vi "Read All Analog Channels.vi"(7 "error in":errorcluster, 9 "Voltage Data":bool=TRUE, 10 "VISA resource name":refnum<visa-resource-name>) -> (0 "error out":errorcluster, 2 "Analog output cluster":T1, 3 "VISA resource name out":refnum<visa-resource-name>)   [LabVIEW 2020, in "BDAQ-6104.lvlib"]
uses:
  <instrlib>/BDAQ-6104/BDAQ-6104.lvlib
panel:
  out "read buffer":string
  in  "AIO Cluster":T1
  out "Volts 0":dbl
  out "Volts 1":dbl
  out "Volts 2":dbl
  out "Volts 3":dbl
  out "Volts 4":dbl
  out "Volts 5":dbl
  out "Value 0":i32
  out "Value 1":i32
  out "Vaolue 2":i32
  out "Value 3":i32
  out "Value 4":i32
  out "Value 5":i32
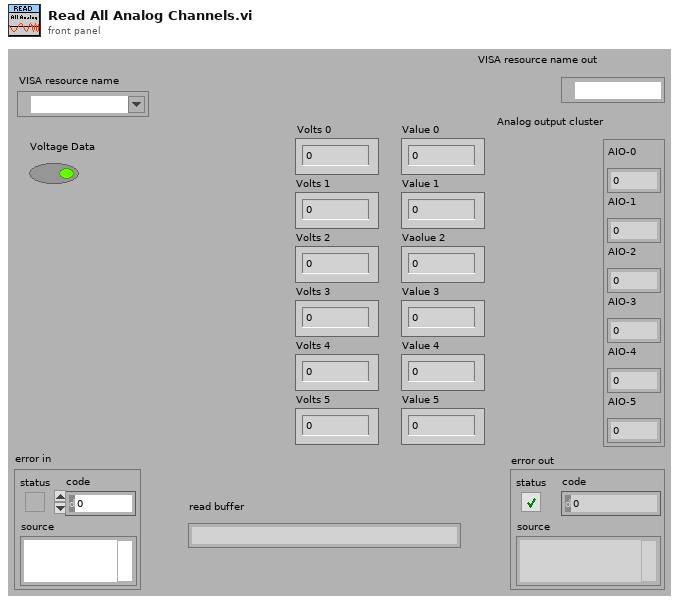
[diagram p1: front panel]
types:
  T1 = cluster{"AIO-0":dbl, "AIO-1":dbl, "AIO-2":dbl, "AIO-3":dbl, "AIO-4":dbl, "AIO-5":dbl}
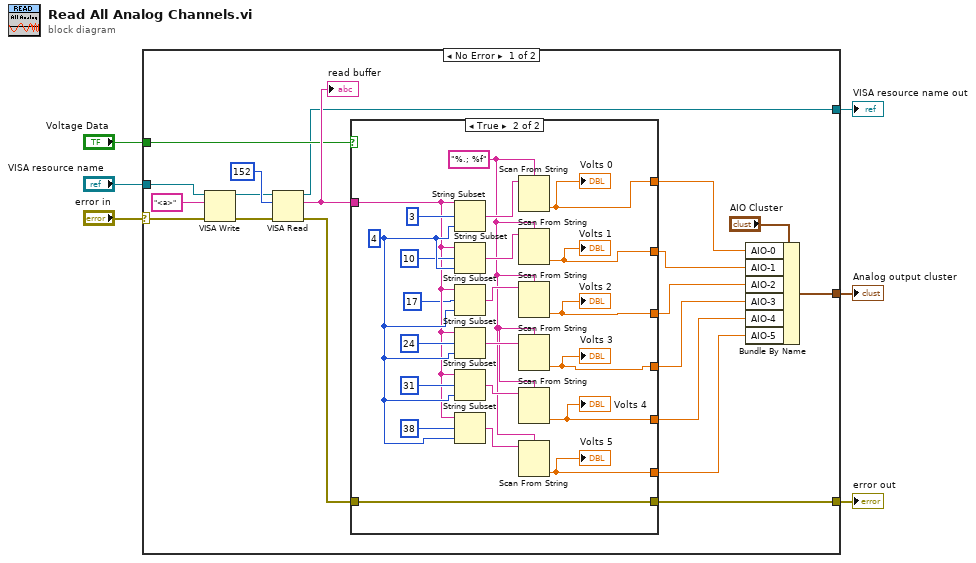
[diagram p0: block diagram]
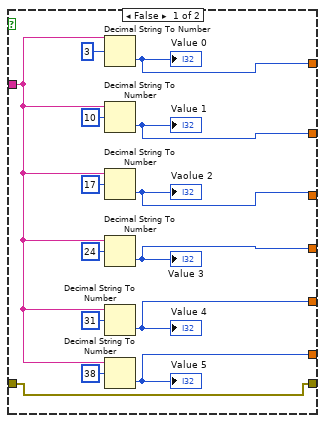
[diagram p2: hidden frame]
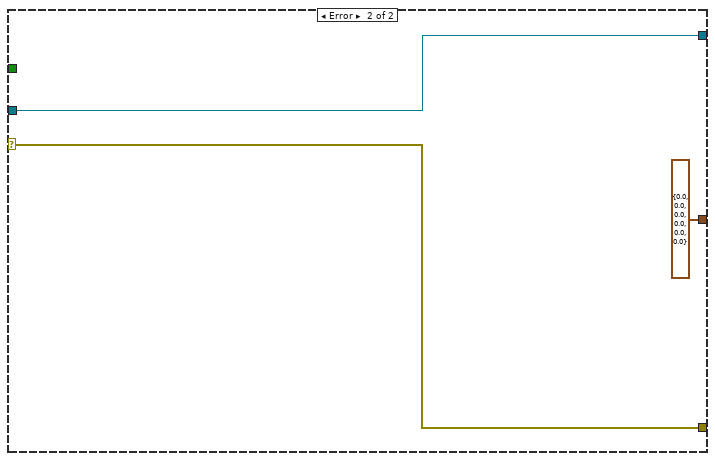
[diagram p3: hidden frame]
diagram:
  n1 = case shown="No Error" "error in" {
    selector: "error in" -> [w7 w63]
    tunnel: "VISA resource name" -> [w24 w64]
    tunnel: [w18 T1 {"AIO-0"=0.0, "AIO-1"=0.0, "AIO-2"=0.0, "AIO-3"=0.0, "AIO-4"=0.0, "AIO-5"=0.0} ("AIO Cluster")] -> w5
    tunnel: [w10 w63] -> w4
    tunnel: "Voltage Data" -> [w9 _]
    tunnel: [w8 w64] -> w2
    frame No Error {
      n2 = VISA Write(VISA resource name=w24, write buffer="<a>", error in (no error)=w7) -> (VISA resource name out=w21:refnum<visa-resource-name>, error out=w23:errorcluster)  [unwired: 1 out]
      n3 = VISA Read(VISA resource name=w21, byte count=u32 152, error in (no error)=w23) -> (VISA resource name out=w8:refnum<visa-resource-name>, read buffer=w20:string, error out=w11:errorcluster)  [unwired: 1 out]
      "read buffer" <- w20
      n4 = case shown="True" w9 {
        tunnel: w20 -> [w33 w55]
        tunnel: [w32 w47] -> w17
        tunnel: [w31 w46] -> w16
        tunnel: [w30 w45] -> w15
        tunnel: [w29 w44] -> w14
        tunnel: [w28 w43] -> w13
        tunnel: [w27 w42] -> w12
        tunnel: w11 -> [w26 w40]
        tunnel: [w26 w40] -> w10
        frame False {
          n5 = Decimal String To Number(string=w33, offset=3) -> (number=w32:i32)  [unwired: 1 in, 1 out]
          "Value 0" <- w32
          n6 = Decimal String To Number(string=w33, offset=10) -> (number=w31:i32)  [unwired: 1 in, 1 out]
          "Value 1" <- w31
          n7 = Decimal String To Number(string=w33, offset=17) -> (number=w30:i32)  [unwired: 1 in, 1 out]
          "Vaolue 2" <- w30
          n8 = Decimal String To Number(string=w33, offset=24) -> (number=w29:i32)  [unwired: 1 in, 1 out]
          "Value 3" <- w29
          n9 = Decimal String To Number(string=w33, offset=31) -> (number=w28:i32)  [unwired: 1 in, 1 out]
          "Value 4" <- w28
          n10 = Decimal String To Number(string=w33, offset=38) -> (number=w27:i32)  [unwired: 1 in, 1 out]
          "Value 5" <- w27
        }
        frame True {
          w48 = "%.; %f" ("format string")
          w60 = 4 ("length (rest)")
          n11 = String Subset(string=w55, offset (0)=3, length (rest)=w60) -> (substring=w54:string)
          n12 = String Subset(string=w55, offset (0)=10, length (rest)=w60) -> (substring=w53:string)
          n13 = String Subset(string=w55, offset (0)=17 ("length (rest)"), length (rest)=w60) -> (substring=w52:string)
          n14 = String Subset(string=w55, offset (0)=24, length (rest)=w60) -> (substring=w51:string)
          n15 = String Subset(string=w55, offset (0)=31, length (rest)=w60) -> (substring=w50:string)
          n16 = String Subset(string=w55, offset (0)=38, length (rest)=w60) -> (substring=w49:string)
          n17 = Scan From String(format string=w48, input string=w54) -> (output 1=w47:dbl)  [unwired: 3 in, 3 out]
          "Volts 0" <- w47
          n18 = Scan From String(format string=w48, input string=w53) -> (output 1=w46:dbl)  [unwired: 3 in, 3 out]
          "Volts 1" <- w46
          n19 = Scan From String(format string=w48, input string=w52) -> (output 1=w45:dbl)  [unwired: 3 in, 3 out]
          "Volts 2" <- w45
          n20 = Scan From String(format string=w48, input string=w51) -> (output 1=w44:dbl)  [unwired: 3 in, 3 out]
          "Volts 3" <- w44
          n21 = Scan From String(format string=w48, input string=w50) -> (output 1=w43:dbl)  [unwired: 3 in, 3 out]
          "Volts 4" <- w43
          n22 = Scan From String(format string=w48, input string=w49) -> (output 1=w42:dbl)  [unwired: 3 in, 3 out]
          "Volts 5" <- w42
        }
      }
      n23 = Bundle By Name(cluster="AIO Cluster", "AIO-0"=w17, "AIO-1"=w16, "AIO-2"=w15, "AIO-3"=w14, "AIO-4"=w13, "AIO-5"=w12) -> (w18:T1)
    }
    frame Error {
    }
  }
  "error out" <- w4
  "Analog output cluster" <- w5
  "VISA resource name out" <- w2
